vi "Find spot in image.vi"(9 "Image":T1) -> (2 "Y Centroid":dbl, 3 "X Centroid":dbl)   [LabVIEW 2012]
uses:
  <vilib>/vision/Image Controls.llb/IMAQ Image.ctl
  <vilib>/vision/NI_Vision_Development_Module.lvlib
  <resource>/objmgr/IMAQImage.rc
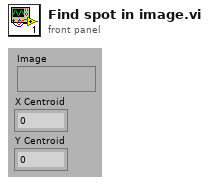
[diagram p1: front panel]
types:
  T1 = typedef "IMAQ Image.ctl" = refnum<image>
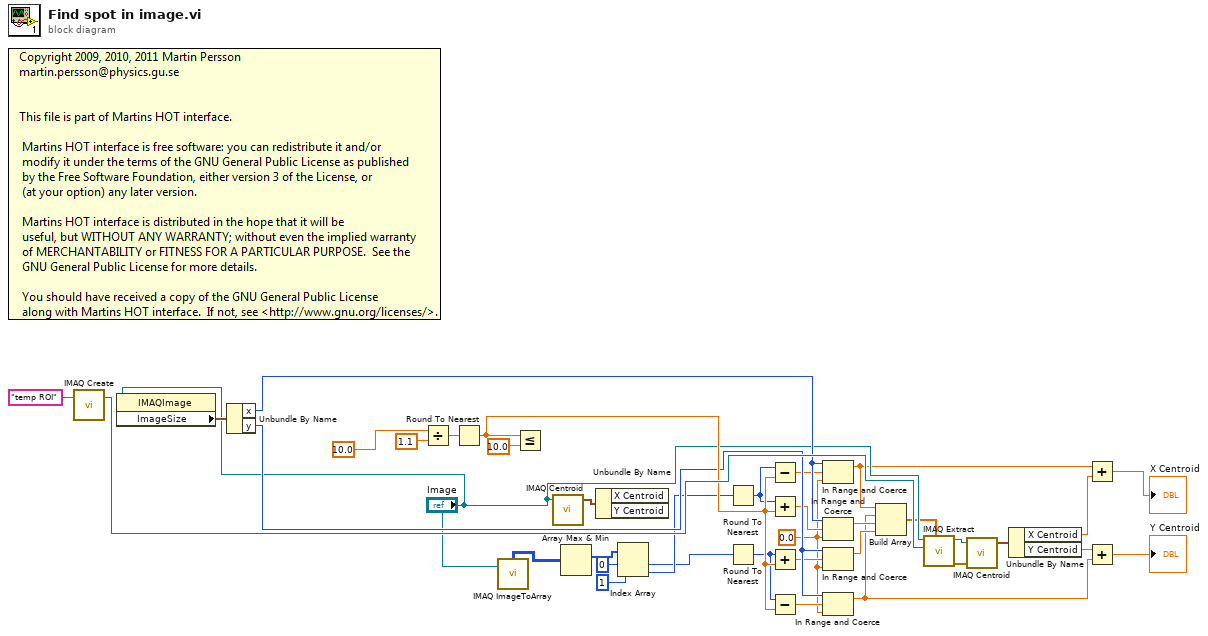
[diagram p0: block diagram]
diagram:
  w4 = 0.0 ("lower limit")
  n1 = call "IMAQ Create"("Image Name"="temp ROI") -> ("New Image"=w35:T1)  [unwired: 4 in, 1 out]
  n2 = property class="IMAQImage"(reference="Image") -> ("ImageSize"=w34:cluster{"x":i32, "y":i32})  [unwired: 1 in, 2 out]
  n3 = Unbundle By Name(w34) -> ("x"=w32:i32, "y"=w31:i32)
  n4 = Divide(x=10.0, y=1.1) -> (x/y=w21:dbl)
  n5 = Round To Nearest(number=w21) -> (nearest integer value=w33:dbl)
  n6 = call "IMAQ ImageToArray"("Image"="Image") -> ("Image Pixels (U8)"=w30:u8[][])  [unwired: 3 in, 4 out]
  n7 = Less Or Equal?(x=w33, y=10.0) -> ()  [unwired: 1 out]
  n8 = call "IMAQ Centroid"("Image"="Image") -> ("Centroid"=w36:cluster{"X Centroid":sgl, "Y Centroid":sgl})  [unwired: 3 in, 1 out]
  n9 = Array Max & Min(array=w30) -> (max index (indices)=w29:i32[])  [unwired: 3 out]
  n10 = Unbundle By Name(w36) -> ()  [unwired: 2 out]
  n11 = Index Array(array=w29, index #1=0 ("index"), index #2=1 ("index")) -> (element #1=w23:i32, element #2=w24:i32)
  n12 = Round To Nearest(number=w24) -> (nearest integer value=w13:i32)
  n13 = Round To Nearest(number=w23) -> (nearest integer value=w12:i32)
  n14 = Subtract(x=w13, y=w33) -> (x-y=w11:dbl)
  n15 = Add(x=w13, y=w33) -> (x+y=w9:dbl)
  n16 = Add(x=w12, y=w33) -> (x+y=w7:dbl)
  n17 = Subtract(x=w12, y=w33) -> (x-y=w5:dbl)
  n18 = In Range and Coerce(upper limit=w32, x=w11, lower limit=w4) -> (coerced(x)=w10:dbl)  [unwired: 1 out]
  n19 = In Range and Coerce(upper limit=w32, x=w9, lower limit=w4) -> (coerced(x)=w8:dbl)  [unwired: 1 out]
  n20 = In Range and Coerce(upper limit=w31, x=w7, lower limit=w4) -> (coerced(x)=w6:dbl)  [unwired: 1 out]
  n21 = In Range and Coerce(upper limit=w31, x=w5, lower limit=w4) -> (coerced(x)=w3:dbl)  [unwired: 1 out]
  n22 = Build Array(w10, w3, w8, w6) -> (w17:dbl[])
  n23 = call "IMAQ Extract"("Optional Rectangle"=w17, "Image Dst"=w35, "Image Src"="Image") -> ("error out"=w19:errorcluster, "Image Dst Out"=w18:T1)  [unwired: 7 in]
  n24 = call "IMAQ Centroid"("error in (no error)"=w19, "Image"=w18) -> ("Centroid"=w16:cluster{"X Centroid":sgl, "Y Centroid":sgl})  [unwired: 2 in, 1 out]
  n25 = Unbundle By Name(w16) -> ("X Centroid"=w15:sgl, "Y Centroid"=w14:sgl)
  n26 = Add(x=w10, y=w15) -> (x+y=→"X Centroid":dbl)
  n27 = Add(x=w14, y=w3) -> (x+y=→"Y Centroid":dbl)
